vi "S2C_ManageRemoteError.vi"(8 "Error In":errorcluster) -> (0 "Error Out":errorcluster)   [LabVIEW 2015]
doc: "Write an error to file, displays the error to the user, and exits the application if warranted."
uses:
  Globals/S2C_Globals.vi
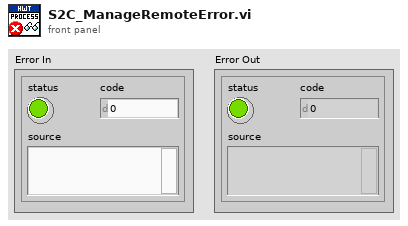
[diagram p1: front panel]
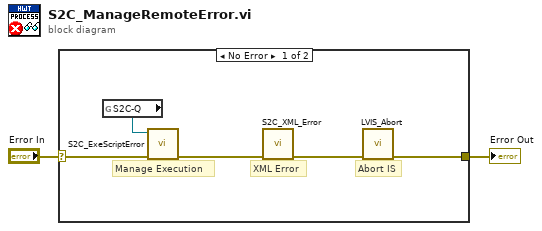
[diagram p0: block diagram]
diagram:
  n1 = case shown="No Error" "Error In" {
    selector: "Error In" -> [w5 w8]
    tunnel: [w6 w8] -> w1
    frame No Error {
      # "XML Error"
      # "Manage Execution"
      # "Abort IS"
      n2 = global read "S2C_Globals.vi" "S2C-Q"() -> (w7:refnum<queue>)
      n3 = call "S2C_ExeScriptError.vi"("Error In"=w5, "Q-Ref"=w7) -> ("Error Out"=w4:errorcluster)  [unwired: 9 in]
      n4 = call "S2C_XML_Error.vi"("Error In"=w4) -> ("Error Out"=w3:errorcluster)  [unwired: 10 in]
      n5 = call "LVIS_Abort.vi"("Error In"=w3) -> ("Error Out"=w6:errorcluster)  [unwired: 10 in]
    }
    frame Error {
    }
  }
  "Error Out" <- w1
